vi "Benchmark exprParser_SubVI.vi"(8 "error in (no error)":errorcluster, 10 "Iterations":i32, 11 "Expression":string) -> (0 "error out":errorcluster, 2 "x":dbl[](array[numeric]), 3 "y":dbl[](array[numeric]), 5 "dt":u32)   [LabVIEW 2015]
uses:
  <vilib>/gmath/NI_Gmath.lvlib
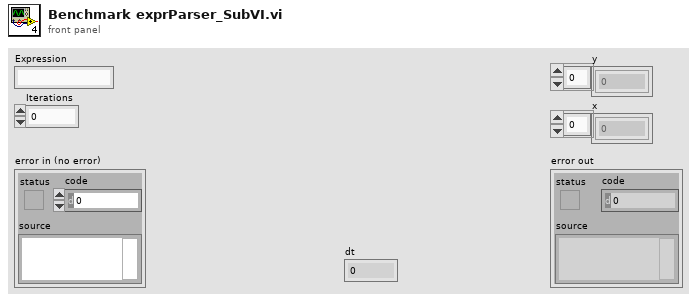
[diagram p1: front panel]
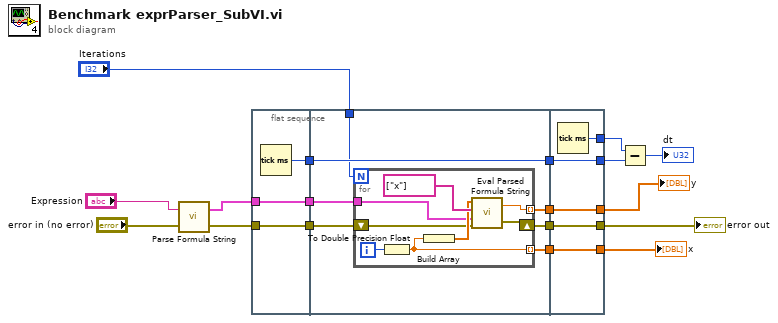
[diagram p0: block diagram]
diagram:
  n1 = call <vilib>:"Parse Formula String.vi"("error in (no error)"="error in (no error)", "formula"="Expression") -> ("error out"=w4:errorcluster, "Parsed Formula"=w2:cluster{"Table":i32[][], "Y Values":dbl[]})
  n2 = flat-sequence {
    tunnel: w4 -> [w20]
    tunnel: w2 -> [w21]
    tunnel: [w21] -> w16
    tunnel: [w20] -> w15
    tunnel: [w19] -> w10
    tunnel: w16 -> [w22]
    tunnel: w15 -> [w28]
    tunnel: [w27] -> w14
    tunnel: [w26] -> w13
    tunnel: [w25] -> w12
    tunnel: [w24] -> w11
    tunnel: w10 -> [w24]
    tunnel: "Iterations" -> [w23]
    tunnel: [w39] -> w17
    tunnel: [w40] -> w18
    tunnel: [w41] -> w1
    tunnel: w14 -> [w41]
    tunnel: w13 -> [w40]
    tunnel: w12 -> [w39]
    tunnel: [w38] -> w8
    tunnel: w11 -> [w38]
    tunnel: [w37] -> w9
    frame #0 {
      n3 = Tick Count (ms)() -> (millisecond timer value=w19:u32)
    }
    frame #1 {
      n4 = for {
        N: w23 -> [_]
        shift-right: [w29] -> w27
        shift-left: w28 -> [w32]
        tunnel: [w31] -> w26 mode=indexing
        tunnel: [w34] -> w25 mode=indexing
        tunnel: w22 -> [w30]
        i -> [w36]
        n5 = To Double Precision Float(number=w36) -> (double precision float=w34:dbl)
        n6 = Build Array(w34) -> (w33:dbl[])
        n7 = call <vilib>:"Eval Parsed Formula String.vi"("error in (no error)"=w32, "Parsed Formula"=w30, "Variables"=string[] ["x"], "X Values"=w33) -> ("error out"=w29:errorcluster, "y value"=w31:dbl)
      }
    }
    frame #2 {
      n8 = Tick Count (ms)() -> (millisecond timer value=w37:u32)
    }
  }
  n9 = Subtract(x=w9, y=w8) -> (x-y=→"dt":u32)
  "y" <- w18
  "x" <- w17
  "error out" <- w1
